vi "Save_Recall Secondary Frame.vi"(0 "VISA Resource Name":refnum<visa-resource-name>, 5 "Modulation Format (0:NADC)":T1(ring), 9 "Action (T:SAVE)":bool=TRUE, 11 "error in (no error)":errorcluster {"code" format="%.0x"}) -> (4 "VISA Resource Name Out":refnum<visa-resource-name>, 15 "error out":errorcluster {"code" format="%.0x"})   [LabVIEW 2012, in "Agilent ESG Series.lvlib"]
doc: "This VI is used to save or recall the secondary frame."
uses:
  <instrlib>/Agilent ESG Series/Agilent ESG Series.lvlib
panel:
  # "SAVE"
  # "RECALL"
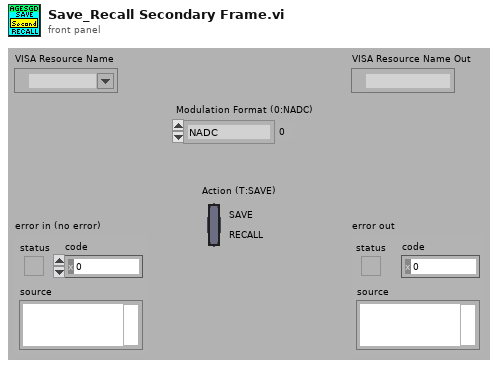
[diagram p1: front panel]
types:
  T1 = enum16{"NADC", "GSM", "PDC", "PHS", "DECT", "TETRA"}
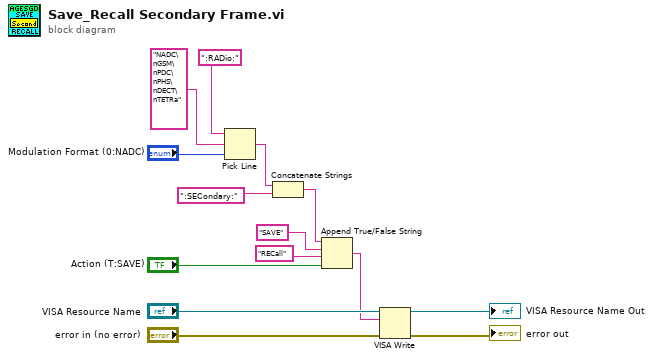
[diagram p0: block diagram]
diagram:
  n1 = Pick Line(string ("")=":RADio:", multi-line string="NADC\nGSM\nPDC\nPHS\nDECT\nTETRa", line index="Modulation Format (0:NADC)") -> (output string=w4:string)
  n2 = Concatenate Strings(w4, ":SECondary:" ("string (\"\")")) -> (w7:string)
  n3 = Append True/False String(1:"Action (T:SAVE)", 2:"RECall" ("false string"), 3:"SAVE" ("true string"), 4:w7) -> (0:w1:string)
  n4 = VISA Write(VISA resource name="VISA Resource Name", write buffer=w1, error in (no error)="error in (no error)") -> (VISA resource name out=→"VISA Resource Name Out":refnum<visa-resource-name>, error out=→"error out":errorcluster)  [unwired: 1 out]
